vi "False.vi"(0 "VI Reference In":refnum<vi>, 1 "Test Label":string, 2 "delimiter (>>)":string=">>", 3 "Assert Only? (F)":bool, 5 "Control Path":string, 11 "Error In":errorcluster, 12 "Assert Interval(10 ms)":u32=10, 13 "Timeout(5 sec)":dbl=5.0) -> (4 "VI Reference Out":refnum<vi>, 6 "Asserted Value":bool, 15 "Error Out":errorcluster)   [LabVIEW 2016, in "Drona.lvlib" / "AssertControlValue.lvlib"]
doc: "Asserts if the value of control is false.\n\nThe input control name is given as a string , incase of path, use delimiters inbetween the path.\nThis VI gets the value of the control, untill the value is false."
uses:
  AssertControlValue.lvlib
  Get/GetControlRef/GetControlRefByPath.vi
  <vilib>/addons/_JKI Toolkits/Caraya/classes/Assert/Assert.lvclass
  Get/GetControlRef/GetControlRef.lvlib
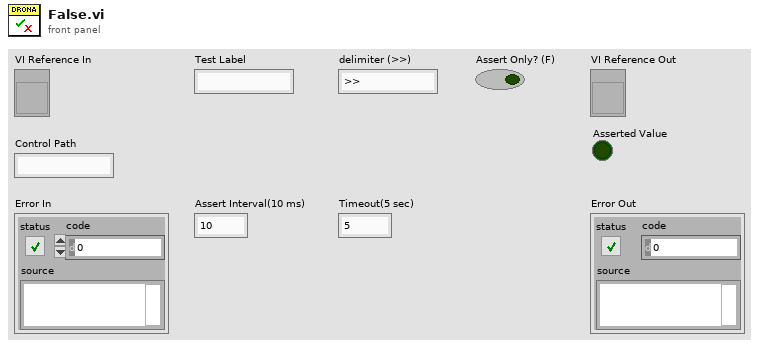
[diagram p1: front panel]
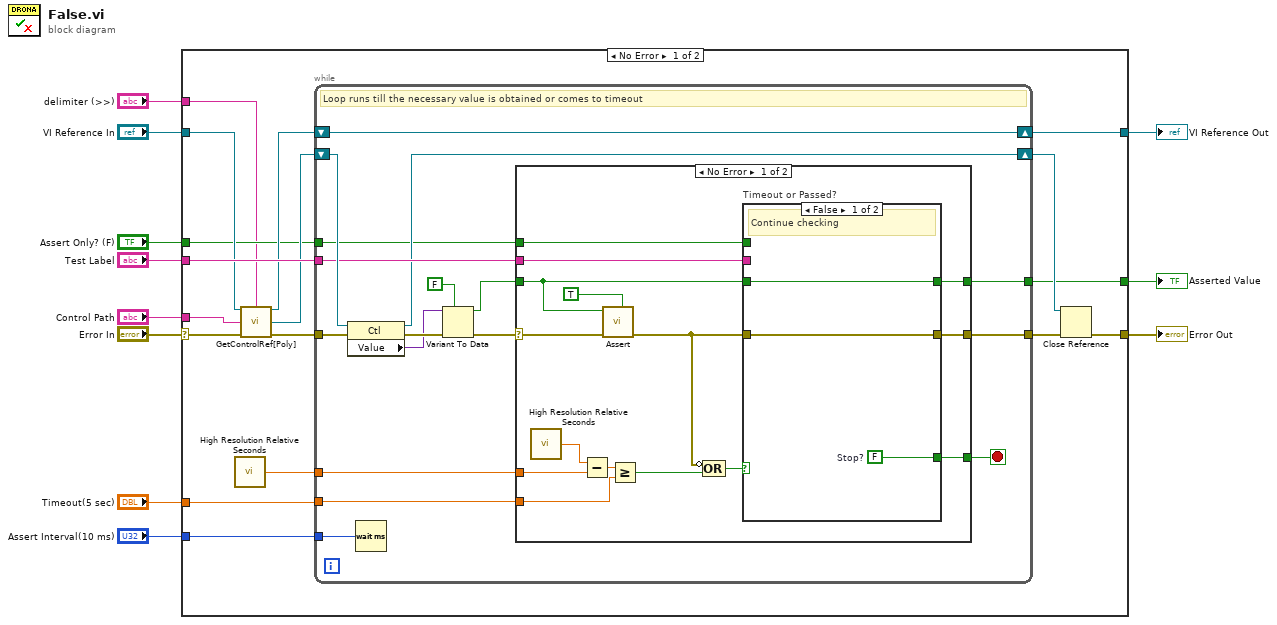
[diagram p0: block diagram]
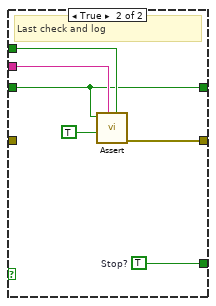
[diagram p2: hidden frame]
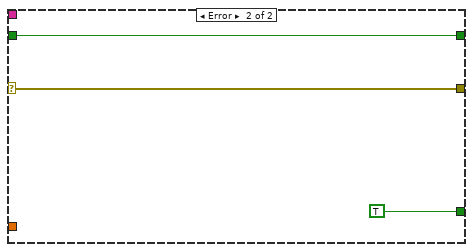
[diagram p3: hidden frame]
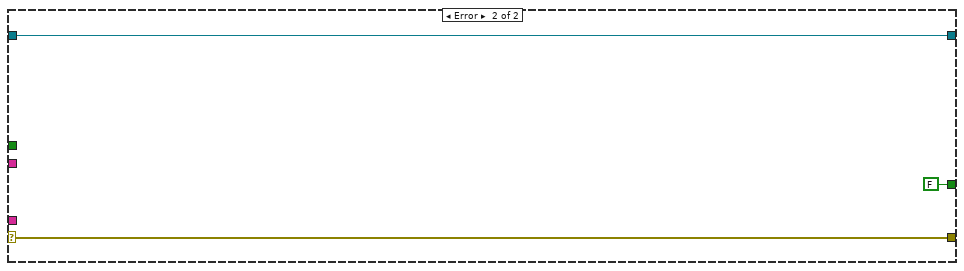
[diagram p4: hidden frame]
diagram:
  n1 = case shown="No Error" "Error In" {
    selector: "Error In" -> [w23 w75]
    tunnel: "Timeout(5 sec)" -> [w28 _]
    tunnel: [w27 w74] -> w10
    tunnel: [w16 w75] -> w9
    tunnel: "Assert Interval(10 ms)" -> [w25 _]
    tunnel: "Test Label" -> [w24 _]
    tunnel: "VI Reference In" -> [w22 w74]
    tunnel: "Control Path" -> [w21 _]
    tunnel: "delimiter (>>)" -> [w12 _]
    tunnel: "Assert Only? (F)" -> [w14 _]
    tunnel: [w13 FALSE] -> w1
    frame No Error {
      n2 = call <vilib>:"High Resolution Relative Seconds.vi"() -> ("relative seconds"=w20:dbl)
      n3 = call-poly "GetControlRef[Poly].vi"("VI Reference In"=w22, "delimiter (>>)"=w12, "Control Path"=w21, "error In"=w23) -> ("VI Reference Out"=w18:refnum<vi>, "Ctl Refnum"=w17:refnum<vi>, "error out"=w19:errorcluster)  [unwired: 9 in]
      n4 = while {
        tunnel: w28 -> [w44]
        tunnel: w20 -> [w45]
        tunnel: w19 -> [w39]
        tunnel: [w42] -> w26
        tunnel: w25 -> [w40]
        tunnel: w24 -> [w36]
        shift-right: [w37] -> w27
        shift-left: w18 -> [w37]
        shift-right: [w35] -> w15
        shift-left: w17 -> [w38]
        tunnel: w14 -> [w30]
        tunnel: [w29] -> w13
        stop <- w43 stop-if-true
        # "Loop runs till the necessary value is obtained or comes to timeout"
        n5 = property class="Ctl"(reference=w38, error in=w39) -> (reference out=w35:refnum<vi>, error out=w41:errorcluster, "Value"=w33:variant)
        n6 = Wait (ms)(milliseconds to wait=w40) -> ()  [unwired: 1 out]
        n7 = Variant To Data(error in=w41, type=FALSE, Variant=w33) -> (data=w32:bool, error out=w34:errorcluster)
        n8 = case shown="No Error" w34 {
          selector: w34 -> [w56 w72]
          tunnel: w45 -> [w60 _]
          tunnel: w44 -> [w57 _]
          tunnel: [w49 TRUE] -> w43
          tunnel: [w50 w72] -> w42
          tunnel: w32 -> [w48 w70]
          tunnel: w36 -> [w55 _]
          tunnel: w30 -> [w47 _]
          tunnel: [w46 w70] -> w29
          frame No Error {
            n9 = call <vilib>:"High Resolution Relative Seconds.vi"() -> ("relative seconds"=w59:dbl)
            n10 = Subtract(x=w59, y=w60) -> (x-y=w58:dbl)
            n11 = call-poly <vilib>:"Assert.vi"("Assert Only? (F)"=TRUE, "error in (no error)"=w56, "False?"=w48) -> ("error out"=w53:errorcluster)  [unwired: 7 in, 1 out]
            n12 = Greater Or Equal?(x=w58, y=w57) -> (x >= y?=w54:bool)
            n13 = Compound Arithmetic op=OR(invert w53, w54) -> (w52:bool)
            n14 = case "Timeout or Passed?" shown="False" w52 {
              tunnel: w53 -> [w63 _]
              tunnel: w48 -> [w61 w64]
              tunnel: w55 -> [_ w69]
              tunnel: [w63 w68] -> w50
              tunnel: [w62 w67] -> w49
              tunnel: w47 -> [_ w65]
              tunnel: [w61 w64] -> w46
              frame False {
                w62 = FALSE  # Stop?
                # "Continue checking"
              }
              frame True {
                w67 = TRUE  # Stop?
                # "Last check and log"
                n15 = call-poly <vilib>:"Assert.vi"("Assert Only? (F)"=w65, "Label"=w69, "Register with caller test (F)"=TRUE, "False?"=w64) -> ("error out"=w68:errorcluster)  [unwired: 6 in, 1 out]
              }
            }
          }
          frame Error {
          }
        }
      }
      n16 = Close Reference(reference=w15, error in (no error)=w26) -> (error out=w16:errorcluster)
    }
    frame Error {
    }
  }
  "Error Out" <- w9
  "VI Reference Out" <- w10
  "Asserted Value" <- w1
